vi "Configure.vi"(8 "error in (no error)":errorcluster, 11 "IMAQdx Camera in":refnum<class "IMAQdx Camera.lvclass">) -> (0 "error out":errorcluster, 3 "IMAQdx Camera out":refnum<class "IMAQdx Camera.lvclass">)   [LabVIEW 2011, in "IMAQdx Camera.lvclass"]
uses:
  IMAQdx Camera.lvclass
  IMAQdx Camera.lvclass/IMAQdx Camera.ctl
  <vilib>/vision/driver/NI_Vision_Acquisition_Software.lvlib
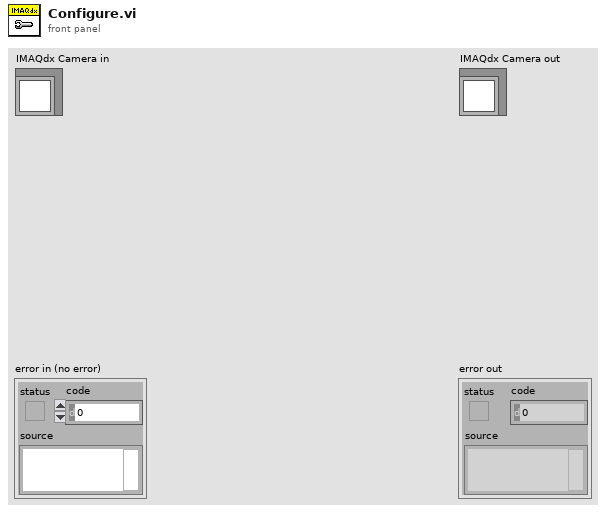
[diagram p1: front panel]
types:
  T1 = typedef "IMAQdx.ctl" = refnum<k21>
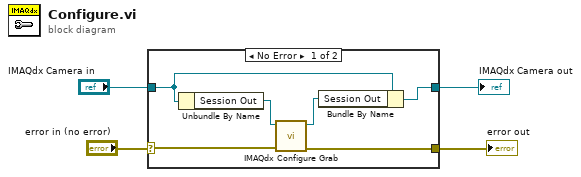
[diagram p0: block diagram]
diagram:
  n1 = case shown="No Error" "error in (no error)" {
    selector: "error in (no error)" -> [w5 w11]
    tunnel: "IMAQdx Camera in" -> [w9 w12]
    tunnel: [w7 w12] -> w3
    tunnel: [w6 w11] -> w2
    frame No Error {
      n2 = Unbundle By Name(w9) -> ("Session Out"=w10:T1)
      n3 = call <vilib>:"IMAQdx Configure Grab.vi"("error in"=w5, "Session In"=w10) -> ("error out"=w6:errorcluster, "Session Out"=w8:T1)  [unwired: 8 in]
      n4 = Bundle By Name(cluster=w9, "Session Out"=w8) -> (w7:refnum<class "IMAQdx Camera.lvclass">)
    }
    frame Error {
    }
  }
  "error out" <- w2
  "IMAQdx Camera out" <- w3
